vi "EGSE Tester.vi"() -> ()   [LabVIEW 2024]
uses:
  <vilib>/Utility/error.llb/DialogType.ctl
  <vilib>/Analysis/baseanly.llb/Mean (DBL).vi
  <instrlib>/Detector SCPI/Detector SCPI.lvlib
  <vilib>/Analysis/NI_AALBase.lvlib
panel:
  out "uS/reading":dbl
  out "Pk-Pk":dbl
  out "mean":dbl format="%0.2f"
  out "Elapsed(uS)":i32
  in  "Gain":u16(ring) items=["High", "Med", "Low"]
  in  "Tab Control":enum32{"PowerMonitor", "ReadADC"}(tab)
  out "Current&Voltage":T1(graph)
  out "Voltage (V)":dbl[](array[numeric])=[3.264, 0.0, 12.488, 12.77]
  out "Current (mA)":dbl[](array[numeric])=[0.0, 0.0, 21.6, -3.65]
  out "Counts":dbl(graph)=160.194
  in  "ResetGraph":bool
  in  "Power":bool
  in  "stop":bool
  in  "Detector":u16(ring) items=["SWIR", "MWIR"]
  in  "DAC Value":i32=2076 min=0 max=4095 step=1
  in  "Oversample":i32=1000 min=1 max=4096
  in  "SPI Clock":i64
  out "Detector Resource":refnum<visa-resource-name>="COM4"
  out "Detector EGSE ID String":string="Aberystwyth University,Enfys Detector,#01,v0.5.0\r\n"
  in  "Detector VISA":refnum<visa-resource-name>="COM4"
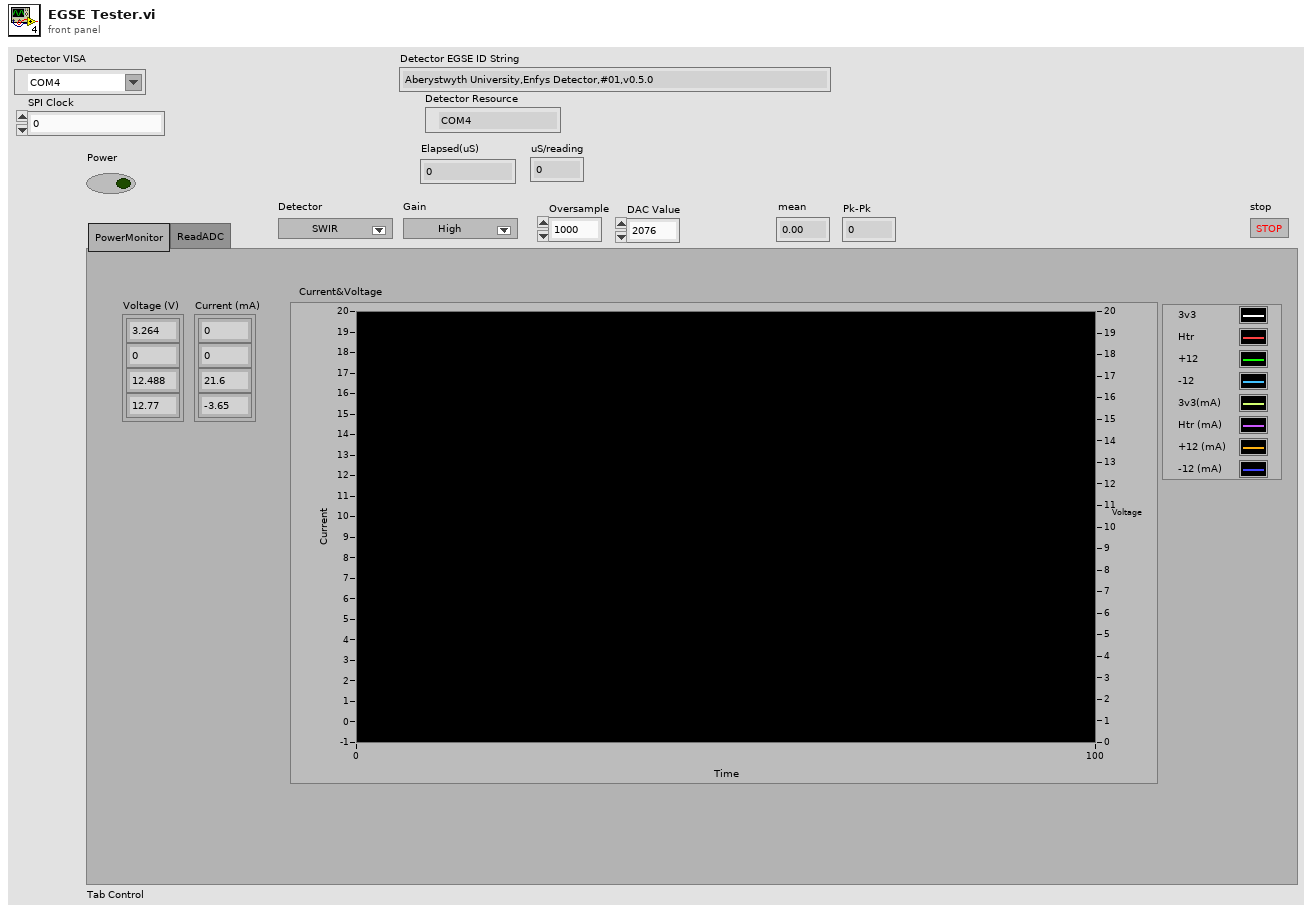
[diagram p1: front panel]
types:
  T1 = cluster{"[0]":dbl, "[1]":dbl, "[2]":dbl, "[3]":dbl, "[4]":dbl, "[5]":dbl, "[6]":dbl, "[7]":dbl, "[8]":dbl}
  T2 = typedef "DialogType.ctl" = u16
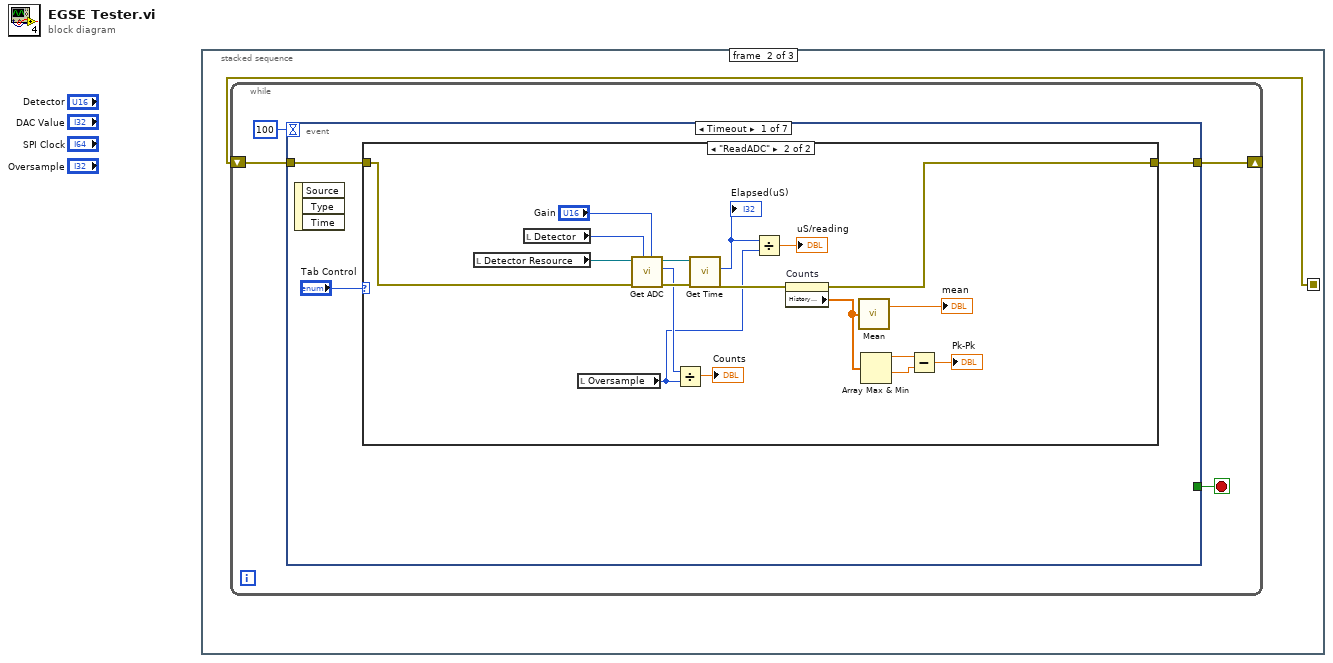
[diagram p0: block diagram]
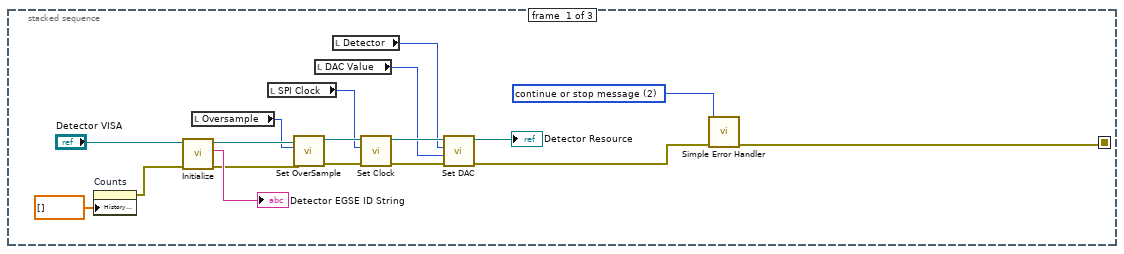
[diagram p2: hidden frame]
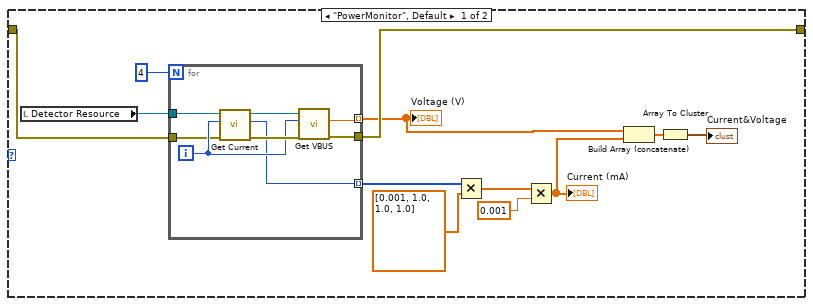
[diagram p3: hidden frame]
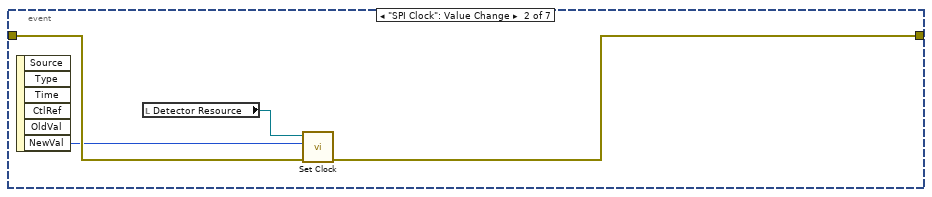
[diagram p4: hidden frame]
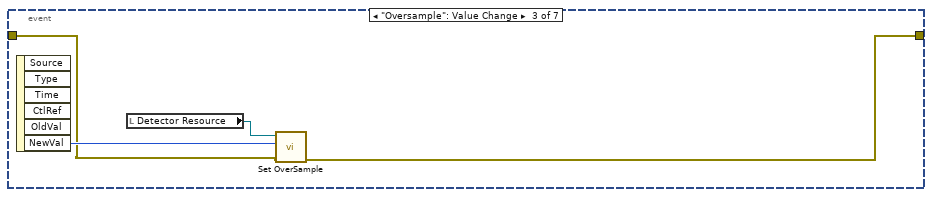
[diagram p5: hidden frame]
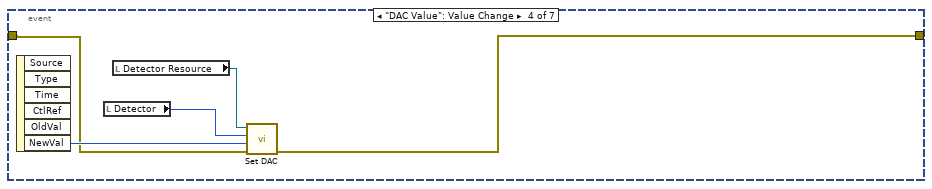
[diagram p6: hidden frame]
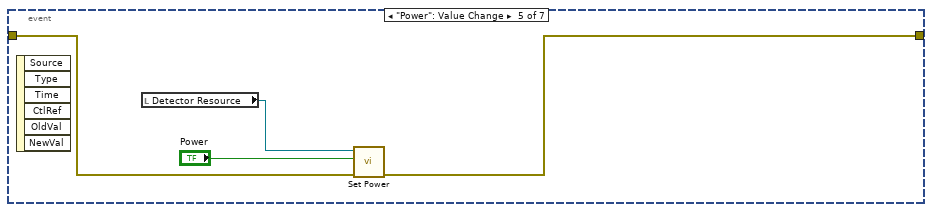
[diagram p7: hidden frame]
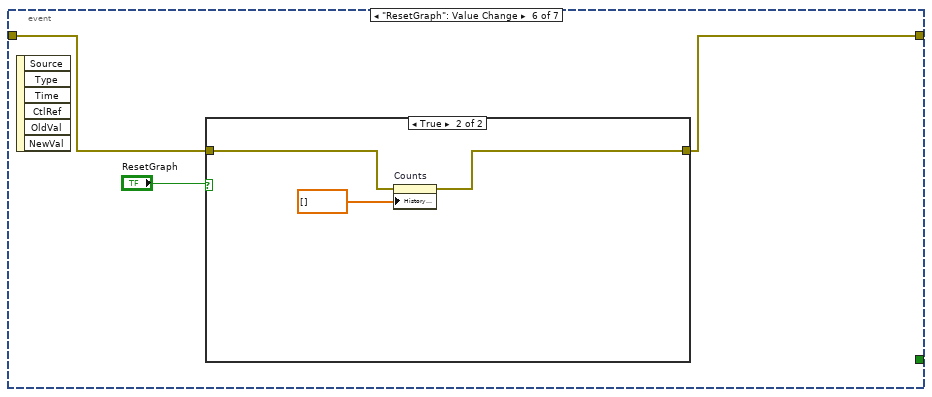
[diagram p8: hidden frame]
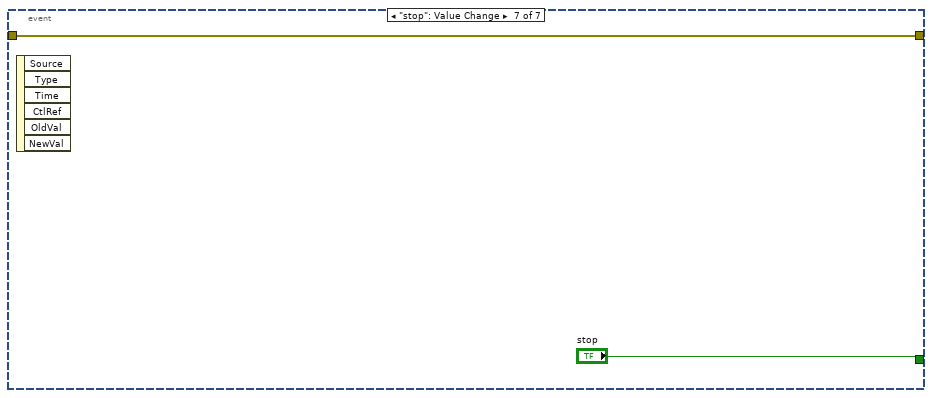
[diagram p10: hidden frame]
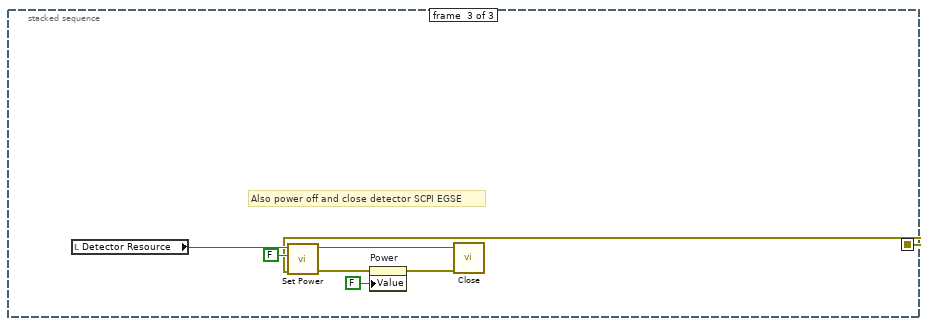
[diagram p11: hidden frame]
diagram:
  n1 = stacked-sequence {
    seq-local: [w3 _ _] -> [_ w19 w91]
    frame #0 {
      w4 = T2 2 items=["no dialog", "OK message", "continue or stop message", "OK message + warnings", "continue/stop + warnings"] ("type of dialog (OK msg:1)")
      n2 = property on="Counts" class="WFChart (strict)"("History Data"=dbl[] []) -> (error out=w2:errorcluster)  [unwired: 2 in, 1 out]
      n3 = call <instrlib>:"Initialize.vi"("error in (no error)"=w2, "VISA resource name"="Detector VISA") -> ("error out"=w15:errorcluster, "ID String"=→"Detector EGSE ID String":string, "VISA resource name out"=w14:refnum<visa-resource-name>)  [unwired: 7 in]
      n4 = local read "Oversample"() -> (w13:i32)
      n5 = local read "SPI Clock"() -> (w8:i64)
      n6 = call <instrlib>:"Set OverSample.vi"("error in (no error)"=w15, "oversample (0)"=w13, "VISA resource name"=w14) -> ("error out"=w12:errorcluster, "VISA resource name out"=w10:refnum<visa-resource-name>)  [unwired: 7 in]
      n7 = local read "DAC Value"() -> (w6:i32)
      n8 = local read "Detector"() -> (w7:u16)
      n9 = call <instrlib>:"Set Clock.vi"("error in (no error)"=w12, "ClockSpeed"=w8, "VISA resource name"=w10) -> ("error out"=w11:errorcluster, "VISA resource name out"=w9:refnum<visa-resource-name>)  [unwired: 7 in]
      n10 = call <instrlib>:"Set DAC.vi"("error in (no error)"=w11, "value (0)"=w6, "chan (0)"=w7, "VISA resource name"=w9) -> ("error out"=w5:errorcluster, "VISA resource name out"=→"Detector Resource":refnum<visa-resource-name>)  [unwired: 6 in]
      n11 = call <vilib>:"Simple Error Handler.vi"("type of dialog (OK msg:1)"=w4, "error in (no error)"=w5) -> ("error out"=w3:errorcluster)  [unwired: 3 in, 4 out]
    }
    frame #1 {
      n12 = while {
        shift-right: [w20] -> _
        shift-left: w19 -> [w21]
        stop <- w22 stop-if-true
        n13 = event shown="[0] Timeout" {
          selector: _ -> [_ _ _ _ _ _ _]
          dyn-events: _ -> [_ _ _ _ _ _ _]
          timeout: 100 -> [_ _ _ _ _ _ _]
          tunnel: [_ _ _ _ _ _ "stop"] -> w22
          tunnel: w21 -> [w26 w68 w71 w76 w79 w83 w89]
          tunnel: [w25 w67 w70 w75 w78 w82 w89] -> w20
          event Timeout {
            n14 = event-data() -> ()  [unwired: 1 in, 3 out]
            n15 = case shown="\"ReadADC\"" "Tab Control" {
              tunnel: w26 -> [w32 w58]
              tunnel: [w31 w56] -> w25
              frame "PowerMonitor", Default {
                n16 = local read "Detector Resource"() -> (w38:refnum<visa-resource-name>)
                n17 = for {
                  N: 4 -> [_]
                  tunnel: w38 -> [w46]
                  tunnel: [w42] -> w36 mode=indexing
                  tunnel: [w41] -> w30 mode=indexing
                  tunnel: w32 -> [w40]
                  tunnel: [w39] -> w31
                  i -> [w43]
                  n18 = call <instrlib>:"Get Current.vi"("error in (no error)"=w40, "chan (1)"=w43, "VISA resource name"=w46) -> ("error out"=w45:errorcluster, "output"=w42:i32, "VISA resource name out"=w44:refnum<visa-resource-name>)  [unwired: 6 in]
                  n19 = call <instrlib>:"Get VBUS.vi"("error in (no error)"=w45, "chan (1)"=w43, "VISA resource name"=w44) -> ("error out"=w39:errorcluster, "output"=w41:dbl)  [unwired: 6 in, 1 out]
                }
                "Voltage (V)" <- w30
                n20 = Multiply(x=w36, y=dbl[] [0.001, 1.0, 1.0, 1.0]) -> (x*y=w34:dbl[])
                n21 = Multiply(x=w34, y=0.001) -> (x*y=w29:dbl[])
                "Current (mA)" <- w29
                n22 = Build Array (concatenate)(w30, w29) -> (w28:dbl[])
                n23 = Array To Cluster(array=w28) -> (cluster=→"Current&Voltage":T1)
              }
              frame "ReadADC" {
                n24 = local read "Detector Resource"() -> (w64:refnum<visa-resource-name>)
                n25 = local read "Detector"() -> (w61:u16)
                n26 = local read "Oversample"() -> (w47:i32)
                n27 = call <instrlib>:"Get ADC.vi"("Gain"="Gain", "Detector"=w61, "error in (no error)"=w58, "VISA resource name"=w64) -> ("error out"=w59:errorcluster, "output"=w49:i32, "VISA resource name out"=w60:refnum<visa-resource-name>)  [unwired: 5 in]
                n28 = Divide(x=w49, y=w47) -> (x/y=→"Counts":dbl)
                n29 = call <instrlib>:"Get Time.vi"("error in (no error)"=w59, "VISA resource name"=w60) -> ("error out"=w57:errorcluster, "output"=w50:i32)  [unwired: 7 in, 1 out]
                "Elapsed(uS)" <- w50
                n30 = Divide(x=w50, y=w47) -> (x/y=→"uS/reading":dbl)
                n31 = property on="Counts" class="WFChart (strict)"(error in=w57) -> (error out=w56:errorcluster, "History Data"=w54:dbl[])  [unwired: 1 in, 1 out]
                n32 = call-poly <vilib>:"Mean.vi"("X"=w54) -> ("mean"=→"mean":dbl)  [unwired: 1 out]
                n33 = Array Max & Min(array=w54) -> (max value=w53:dbl, min value=w52:dbl)  [unwired: 2 out]
                n34 = Subtract(x=w53, y=w52) -> (x-y=→"Pk-Pk":dbl)
              }
            }
          }
          event "SPI Clock": Value Change {
            n35 = event-data() -> ("NewVal"=w65:i64)  [unwired: 1 in, 5 out]
            n36 = local read "Detector Resource"() -> (w66:refnum<visa-resource-name>)
            n37 = call <instrlib>:"Set Clock.vi"("error in (no error)"=w68, "ClockSpeed"=w65, "VISA resource name"=w66) -> ("error out"=w67:errorcluster)  [unwired: 7 in, 1 out]
          }
          event "Oversample": Value Change {
            n38 = event-data() -> ("NewVal"=w72:i32)  [unwired: 1 in, 5 out]
            n39 = local read "Detector Resource"() -> (w69:refnum<visa-resource-name>)
            n40 = call <instrlib>:"Set OverSample.vi"("error in (no error)"=w71, "oversample (0)"=w72, "VISA resource name"=w69) -> ("error out"=w70:errorcluster)  [unwired: 7 in, 1 out]
          }
          event "DAC Value": Value Change {
            n41 = event-data() -> ("NewVal"=w77:i32)  [unwired: 1 in, 5 out]
            n42 = local read "Detector"() -> (w73:u16)
            n43 = local read "Detector Resource"() -> (w74:refnum<visa-resource-name>)
            n44 = call <instrlib>:"Set DAC.vi"("error in (no error)"=w76, "value (0)"=w77, "chan (0)"=w73, "VISA resource name"=w74) -> ("error out"=w75:errorcluster)  [unwired: 6 in, 1 out]
          }
          event "Power": Value Change {
            n45 = event-data() -> ()  [unwired: 1 in, 6 out]
            n46 = local read "Detector Resource"() -> (w80:refnum<visa-resource-name>)
            n47 = call <instrlib>:"Set Power.vi"("error in (no error)"=w79, "Power (0)"="Power", "VISA resource name"=w80) -> ("error out"=w78:errorcluster)  [unwired: 7 in, 1 out]
          }
          event "ResetGraph": Value Change {
            n48 = event-data() -> ()  [unwired: 1 in, 6 out]
            n49 = case shown="True" "ResetGraph" {
              tunnel: w83 -> [w85 w88]
              tunnel: [w85 w87] -> w82
              frame False {
              }
              frame True {
                n50 = property on="Counts" class="WFChart (strict)"(error in=w88, "History Data"=dbl[] []) -> (error out=w87:errorcluster)  [unwired: 1 in, 1 out]
              }
            }
          }
          event "stop": Value Change {
            n51 = event-data() -> ()  [unwired: 1 in, 6 out]
          }
        }
      }
    }
    frame #2 {
      # "Also power off and close detector SCPI EGSE"
      n52 = local read "Detector Resource"() -> (w95:refnum<visa-resource-name>)
      n53 = call <instrlib>:"Set Power.vi"("error in (no error)"=w91, "Power (0)"=FALSE, "VISA resource name"=w95) -> ("error out"=w97:errorcluster, "VISA resource name out"=w94:refnum<visa-resource-name>)  [unwired: 7 in]
      n54 = property on="Power" class="Bool (strict)"(error in=w97, "Value"=FALSE ("Power")) -> (error out=w96:errorcluster)  [unwired: 1 in, 1 out]
      n55 = call <instrlib>:"Close.vi"("error in (no error)"=w96, "VISA resource name"=w94) -> ()  [unwired: 9 in, 1 out]
    }
  }
